vi "Compound.vi"(8 "error in (no error)":errorcluster, 10 "Timespan":u32, 11 "AInterestAccount in":refnum<class "AInterestAccount.lvclass">) -> (0 "error out":errorcluster, 3 "AInterestAccount out":refnum<class "AInterestAccount.lvclass">)   [LabVIEW 2020, in "AInterestAccount.lvclass"]
uses:
  AInterestAccount.lvclass
  AInterestAccount.lvclass/AInterestAccount.ctl
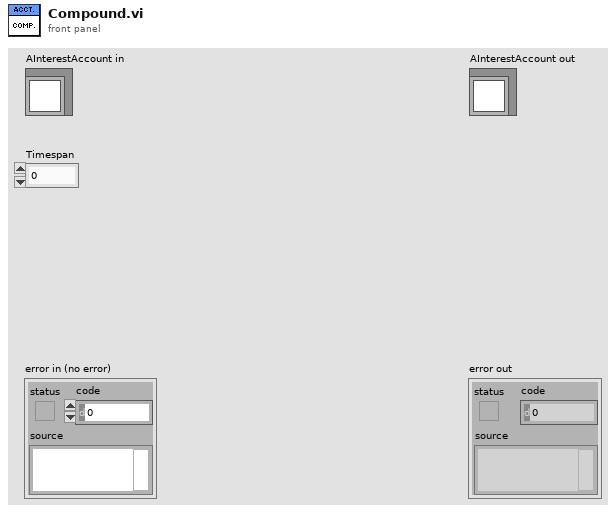
[diagram p1: front panel]
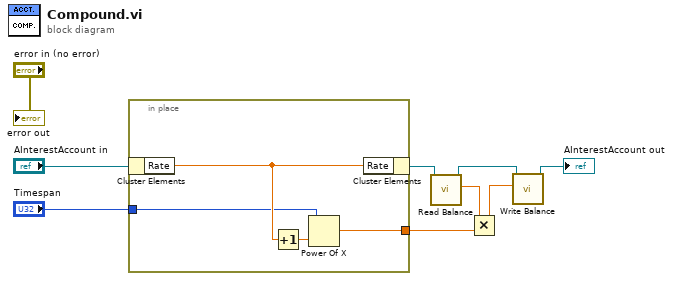
[diagram p0: block diagram]
diagram:
  n1 = in-place {
    in-place-border: "Timespan" -> [w10]
    in-place-border: [w11] -> w3
    n2 = in-place-cluster #1("AInterestAccount in") -> ("Rate"=w13:dbl)
    n3 = Increment(x=w13) -> (x+1=w12:dbl)
    n4 = Power Of X(1:w12, 2:w10) -> (0:w11:dbl)
    n5 = in-place-cluster #1("Rate"=w13) -> (w7:refnum<class "AInterestAccount.lvclass">)
  }
  n6 = call-dynamic "Read Balance.vi"("AAccount in"=w7) -> ("Balance"=w4:dbl, "AAccount out"=w6:refnum<class "AInterestAccount.lvclass">)  [unwired: 8 in, 1 out]
  n7 = Multiply(x=w4, y=w3) -> (x*y=w2:dbl)
  n8 = call-dynamic "Write Balance.vi"("Balance"=w2, "AAccount in"=w6) -> ("AAccount out"=→"AInterestAccount out":refnum<class "AInterestAccount.lvclass">)  [unwired: 8 in, 1 out]
  "error out" <- "error in (no error)"
